vi "temptest2.vi"() -> ()   [LabVIEW 2024]
uses:
  <vilib>/Instr/_visa.llb/VISA Configure Serial Port (Instr).vi
panel:
  in  "FALSE to stop":bool
  out "Heater status 4":bool
  out "Heater status 3":bool
  out "Heater status 2":bool
  out "Heater status":bool
  in  "Setpoint 4":dbl
  in  "Setpoint 3":dbl
  in  "Setpoint 2":dbl
  in  "Setpoint 1":dbl
  out "temp1":dbl
  out "temp2":dbl
  out "temp3":dbl
  out "temp4":dbl
  out "Direct Output":string
  out "error out":errorcluster
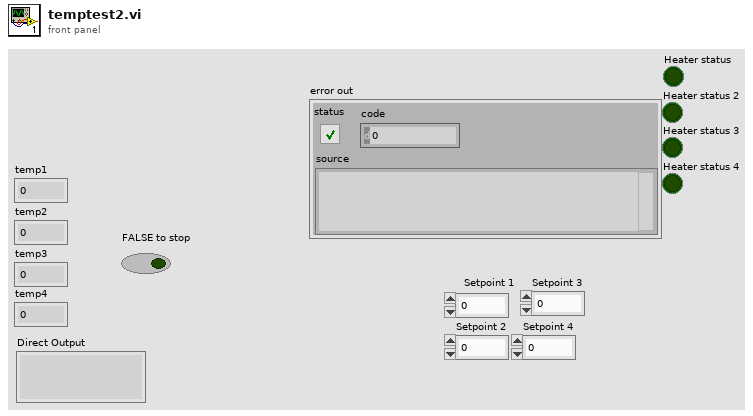
[diagram p1: front panel]
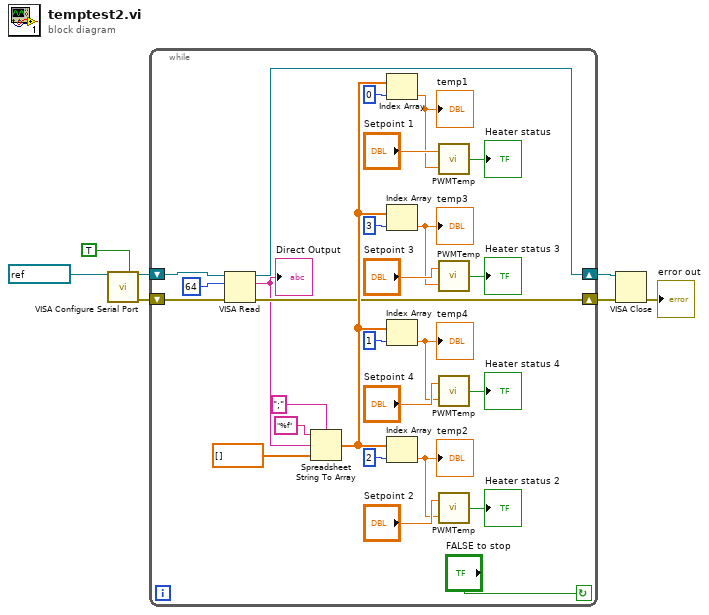
[diagram p0: block diagram]
diagram:
  n1 = call-poly "VISA Configure Serial Port"("VISA resource name"=refnum<visa-resource-name> "COM5", "Enable Termination\nChar (T)"=TRUE ("Enable Termination\nChar (T)")) -> ("VISA resource name out"=w6:refnum<visa-resource-name>, "error out"=w5:errorcluster)  [unwired: 12 in]
  n2 = while {
    shift-right: [w21] -> w4
    shift-left: w6 -> [w25]
    shift-right: [w23] -> w3
    shift-left: w5 -> [w24]
    stop <- "FALSE to stop" continue-if-true
    n3 = VISA Read(VISA resource name=w25, byte count=u32 64, error in (no error)=w24) -> (VISA resource name out=w21:refnum<visa-resource-name>, read buffer=w22:string, error out=w23:errorcluster)  [unwired: 1 out]
    "Direct Output" <- w22
    n4 = Spreadsheet String To Array(delimiter (Tab)=";", format string="%f", spreadsheet string=w22, array type (2D Dbl)=dbl[] []) -> (array=w27:dbl[])
    n5 = Index Array(array=w27, index=0) -> (element=w19:dbl)
    "temp1" <- w19
    n6 = Index Array(array=w27, index=3) -> (element=w12:dbl)
    "temp3" <- w12
    n7 = Index Array(array=w27, index=1) -> (element=w10:dbl)
    "temp4" <- w10
    n8 = Index Array(array=w27, index=2) -> (element=w16:dbl)
    "temp2" <- w16
    n9 = call "PWMTemp.vi"("process variable"=w19, "setpoint"="Setpoint 1") -> ("Heater status"=→"Heater status":bool)
    n10 = call "PWMTemp.vi"("process variable"=w12, "setpoint"="Setpoint 3") -> ("Heater status"=→"Heater status 3":bool)
    n11 = call "PWMTemp.vi"("process variable"=w10, "setpoint"="Setpoint 4") -> ("Heater status"=→"Heater status 4":bool)
    n12 = call "PWMTemp.vi"("process variable"=w16, "setpoint"="Setpoint 2") -> ("Heater status"=→"Heater status 2":bool)
  }
  n13 = VISA Close(VISA resource name=w4, error in (no error)=w3) -> (error out=→"error out":errorcluster)
